vi "Teleop.vi"(0 "Call Context":T2, 1 "Match Info":T1={"Autonomous Elapsed Seconds"=0.0, "TeleOp Elapsed Seconds"=0.0, "Disabled Elapsed Seconds"=0.0, "Visited Autonomous"=FALSE, "Visited TeleOp"=FALSE, "Visited Disabled"=FALSE, "Autonomous Settings"={"Autonomous Style"=enum."Independent", "VI Refnum"=refnum}}) -> ()   [LabVIEW 2011]
doc: "This VI is called for each TeleOp packet received from the DS where the robot is not disabled. It is often used to read from the joysticks and update I/O or to update setpoints for timed control loops. It should complete and return within 20 milliseconds or it may miss DS packets."
uses:
  <vilib>/Rock Robotics/WPI/DriverStation/WPI_DriverStationDerivedRobotMode.ctl
  <vilib>/Rock Robotics/WPI/DriverStation/WPI_DriverStationMatch Info.ctl
  Robot Global Data.vi
  <vilib>/Rock Robotics/WPI/RobotDrive/WPI_RobotDriveArcadeDrive_Standard(NoSaturation).vi
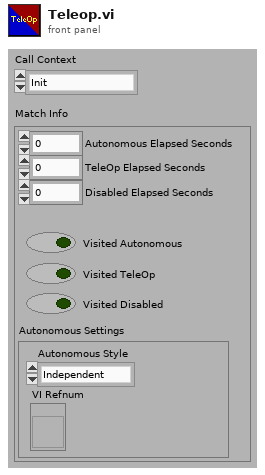
[diagram p1: front panel]
types:
  T1 = typedef "WPI_DriverStationMatch Info.ctl" = cluster{"Autonomous Elapsed Seconds":dbl, "TeleOp Elapsed Seconds":dbl, "Disabled Elapsed Seconds":dbl, "Visited Autonomous":bool, "Visited TeleOp":bool, "Visited Disabled":bool, "Autonomous Settings":cluster{"Autonomous Style":enum16{"Iterative", "Independent"}, "VI Refnum":refnum<vi>}}
  T2 = typedef "WPI_DriverStationDerivedRobotMode.ctl" = enum16{"Init", "Execute", "Stop"}
  T3 = typedef "WPI_JoystickDevRef.ctl" = cluster{"Device":T4}
  T4 = typedef "WPI_JoystickDeviceEnum.ctl" = enum16{"USB 1", "USB 2", "USB 3", "USB 4", "Kinect 1", "Kinect 2"}
  T5 = typedef "WPI_JoystickButtonState.ctl" = cluster{"Button 1":bool, "Button 2":bool, "Button 3":bool, "Button 4":bool, "Button 5":bool, "Button 6":bool, "Button 7":bool, "Button 8":bool, "Button 9":bool, "Button 10":bool, "Button 11":bool, "Button 12":bool}
  T6 = cluster{"axis 1 (x)":dbl, "axis 2 (y)":dbl, "axis 3 (throttle)":dbl, "axis 4":dbl, "axis 5":dbl, "axis 6":dbl}
  T7 = typedef "WPI_RobotDriveDevRef.ctl" = cluster{"DevStatus":errorcluster, "Motors[]":T8[], "Square Inputs":bool, "Max Output":dbl, "Isochronous":bool}
  T8 = typedef "WPI_MotorControlDeviceRef.ctl" = cluster{"DeviceStatus":errorcluster, "Type":enum16{"PWM", "CAN"}, "PWM":cluster{"Digital Module":T9, "PWM Channel":T10, "DeadBand":T11}, "CAN":cluster{"Device Number":u8, "Control Mode":T12, "Semaphore":T13, "Max Vout":dbl}, "Invert":bool, "TransformRef":T14, "InvTransformRef":T14}
  T9 = typedef "FPGA_TypedefDigitalModule.ctl" = enum16{"Digital Module 1", "Digital Module 2"}
  T10 = typedef "FPGA_DIOPWMChannel.ctl" = enum8{"PWM 1", "PWM 2", "PWM 3", "PWM 4", "PWM 5", "PWM 6", "PWM 7", "PWM 8", "PWM 9", "PWM 10", "Invalid"}
  T11 = typedef "WPI_PWMDeadband.ctl" = cluster{"Name":string, "maxPositivePwm":i32, "minPositivePwm":i32, "centerPwm":i32, "maxNegativePwm":i32, "minNegativePwm":i32, "angularRange":u16}
  T12 = typedef "WPI_CANJaguar_ControlMode.ctl" = enum8{"Percent VBus", "Current", "Speed", "Position", "Voltage"}
  T13 = typedef "Semaphore RefNum" = refnum<k1>
  T14 = typedef "WPI_PWMTransform_ConPane.ctl" = refnum<vi>
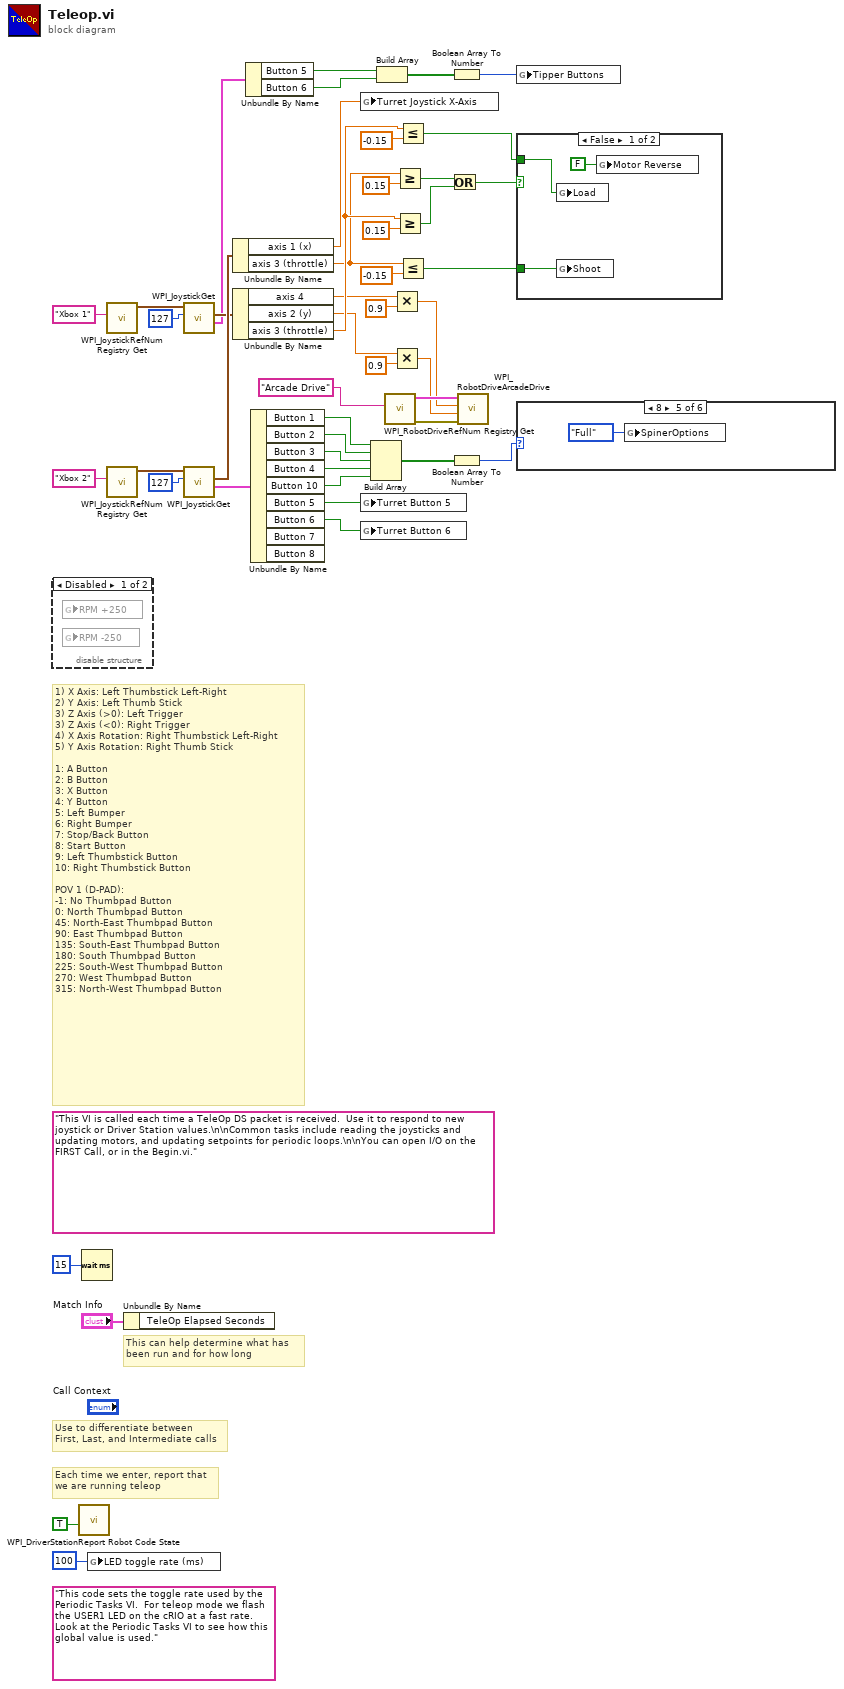
[diagram p0: block diagram]
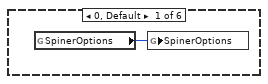
[diagram p3: hidden frame]
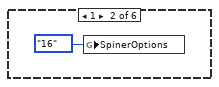
[diagram p4: hidden frame]
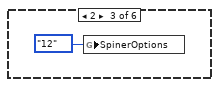
[diagram p5: hidden frame]
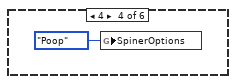
[diagram p6: hidden frame]
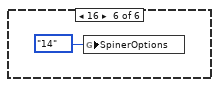
[diagram p7: hidden frame]
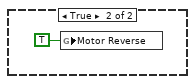
[diagram p8: hidden frame]
diagram:
  (unwired) "This code sets the toggle rate used by the Periodic Tasks VI.  For teleop mode we flash the USER1 LED on the cRIO at a fast rate.  Look at the Periodic Tasks VI to see how this global value is used."
  (unwired) "This VI is called each time a TeleOp DS packet is received.  Use it to respond to new joystick or Driver Station values.\n\nCommon tasks include reading the joysticks and updating motors, and updating setpoints for periodic loops.\n\nYou can open I/O on the FIRST Call, or in the Begin.vi."
  # "1) X Axis: Left Thumbstick Left-Right\n2) Y Axis: Left Thumb Stick\n3) Z Axis (>0): Left Trigger\n3) Z Axis (<0): Right Trigger\n4) X Axis Rotation: Right Thumbstick Left-Right\n5) Y Axis Rotation: Right Thumb Stick\n\n1: A Button\n2: B Button\n3: X Button\n4: Y Button\n5: Left Bumper\n6: Right Bumper\n7: Stop/Back Button\n8: Start Button\n9: Left Thumbstick Button\n10: Right Thumbstick Button\n\nPOV 1 (D-PAD):\n-1: No Thumbpad Button\n0: North Thumbpad Button\n45: North-East Thumbpad Button\n90: East Thumbpad Button\n135: South-East Thumbpad Button\n180: South Thumbpad Button\n225: South-West Thumbpad Button\n270: West Thumbpad Button\n315: North-West Thumbpad Button"
  # "Each time we enter, report that\nwe are running teleop"
  # "Use to differentiate between\nFirst, Last, and Intermediate calls"
  # "This can help determine what has\nbeen run and for how long"
  n1 = disable-structure shown="Disabled" {
    frame Disabled {
      n2 = global read "Robot Global Data.vi" "RPM +250"() -> ()  [unwired: 1 in]
      n3 = global read "Robot Global Data.vi" "RPM -250"() -> ()  [unwired: 1 in]
    }
    frame Enabled {
    }
  }
  n4 = call <vilib>:"WPI_DriverStationReport Robot Code State.vi"("TeleOp"=TRUE ("Autonomous")) -> ()  [unwired: 10 in, 1 out]
  n5 = Wait (ms)(milliseconds to wait=u32 15) -> ()  [unwired: 1 out]
  n6 = global write "Robot Global Data.vi" "LED toggle rate (ms)"(u32 100 ("LED ms toggle rate")) -> ()
  n7 = call <vilib>:"WPI_JoystickRefNum Registry Get.vi"("refnum name"="Xbox 1") -> ("JoystickDevRef"=w44:T3)  [unwired: 9 in, 1 out]
  n8 = call <vilib>:"WPI_JoystickRefNum Registry Get.vi"("refnum name"="Xbox 2") -> ("JoystickDevRef"=w41:T3)  [unwired: 1 in, 9 out]
  n9 = Unbundle By Name("Match Info") -> ()  [unwired: 1 out]
  n10 = call <vilib>:"WPI_JoystickGet.vi"("Scaler"=i8 127, "JoystickDevRef"=w44) -> ("Buttons"=w22:T5, "Axes"=w25:T6)  [unwired: 4 out]
  n11 = call <vilib>:"WPI_JoystickGet.vi"("Scaler"=i8 127, "JoystickDevRef"=w41) -> ("Buttons"=w32:T5, "Axes"=w43:T6)  [unwired: 4 out]
  n12 = Unbundle By Name(w43) -> ("axis 1 (x)"=w35:dbl, "axis 3 (throttle)"=w2:dbl)
  n13 = Unbundle By Name(w25) -> ("axis 4"=w9:dbl, "axis 2 (y)"=w7:dbl, "axis 3 (throttle)"=w18:dbl)
  n14 = Unbundle By Name(w22) -> ("Button 5"=w17:bool, "Button 6"=w16:bool)
  n15 = Unbundle By Name(w32) -> ("Button 1"=w31:bool, "Button 2"=w30:bool, "Button 3"=w29:bool, "Button 4"=w28:bool, "Button 10"=w13:bool, "Button 5"=w26:bool, "Button 6"=w12:bool)  [unwired: 2 out]
  n16 = global write "Robot Global Data.vi" "Turret Joystick X-Axis"(w35) -> ()
  n17 = global write "Robot Global Data.vi" "Turret Button 5"(w26) -> ()
  n18 = global write "Robot Global Data.vi" "Turret Button 6"(w12) -> ()
  n19 = Build Array(w31, w30, w29, w28, w13) -> (w27:bool[])
  n20 = Build Array(w17, w16) -> (w14:bool[])
  n21 = call <vilib>:"WPI_RobotDriveRefNum Registry Get.vi"("refnum name"="Arcade Drive") -> ("error out"=w39:errorcluster, "RobotDriveDevRef"=w40:T7)  [unwired: 9 in]
  n22 = Multiply(x=w9, y=0.9) -> (x*y=w8:dbl)
  n23 = Multiply(x=w7, y=0.9) -> (x*y=w6:dbl)
  n24 = Greater Or Equal?(x=w2, y=0.15) -> (x >= y?=w1:bool)
  n25 = Greater Or Equal?(x=w18, y=0.15) -> (x >= y?=w4:bool)
  n26 = Less Or Equal?(x=w18, y=-0.15) -> (x <= y?=w20:bool)
  n27 = Less Or Equal?(x=w2, y=-0.15) -> (x <= y?=w23:bool)
  n28 = Or(x=w1, y=w4) -> (x .or. y?=w5:bool)
  n29 = Boolean Array To Number(Boolean array=w14) -> (number=w15:u32)
  n30 = Boolean Array To Number(Boolean array=w27) -> (number=w38:u32)
  n31 = call-poly <vilib>:"WPI_RobotDriveArcadeDrive.vi"("error in (no error)"=w39, "Y axis value"=w6, "X axis value"=w8, "RobotDriveDevRef"=w40) -> ()  [unwired: 6 in, 2 out]
  n32 = global write "Robot Global Data.vi" "Tipper Buttons"(w15) -> ()
  n33 = case shown="False" w5 {
    tunnel: w23 -> [w50 _]
    tunnel: w20 -> [w49 _]
    frame False {
      n34 = global write "Robot Global Data.vi" "Load"(w49) -> ()
      n35 = global write "Robot Global Data.vi" "Shoot"(w50) -> ()
      n36 = global write "Robot Global Data.vi" "Motor Reverse"(FALSE ("Motor Reverse")) -> ()
    }
    frame True {
      n37 = global write "Robot Global Data.vi" "Motor Reverse"(TRUE ("Motor Reverse")) -> ()
    }
  }
  n38 = case shown="8" w38 {
    frame 0, Default {
      n39 = global read "Robot Global Data.vi" "SpinerOptions"() -> (w53:enum16{"Full", "16", "14", "12", "Poop"})
      n40 = global write "Robot Global Data.vi" "SpinerOptions"(w53) -> ()
    }
    frame 1 {
      n41 = global write "Robot Global Data.vi" "SpinerOptions"(enum16{"Full", "16", "14", "12", "Poop"}."16" ("SpinerOptions")) -> ()
    }
    frame 2 {
      n42 = global write "Robot Global Data.vi" "SpinerOptions"(enum16{"Full", "16", "14", "12", "Poop"}."12" ("SpinerOptions")) -> ()
    }
    frame 4 {
      n43 = global write "Robot Global Data.vi" "SpinerOptions"(enum16{"Full", "16", "14", "12", "Poop"}."Poop" ("SpinerOptions")) -> ()
    }
    frame 8 {
      n44 = global write "Robot Global Data.vi" "SpinerOptions"(enum16{"Full", "16", "14", "12", "Poop"}."Full" ("SpinerOptions")) -> ()
    }
    frame 16 {
      n45 = global write "Robot Global Data.vi" "SpinerOptions"(enum16{"Full", "16", "14", "12", "Poop"}."14" ("SpinerOptions")) -> ()
    }
  }
